vi "Remove Test Property.vi"(6 "timeout (ms)":i32=-1, 8 "error in (no error)":errorcluster, 10 "testPropertyName":string, 11 "FlexLogger_gRPCAPI in":refnum<class "FlexLogger_gRPC.lvclass">) -> (0 "error out":errorcluster, 3 "FlexLogger_gRPCAPI out":refnum<class "FlexLogger_gRPC.lvclass">)   [LabVIEW 2020, in "FlexLogger_gRPC.lvlib" / "FlexLogger_gRPC.lvclass"]
doc: "Removes a specific test property of currently opened project in flexlogger"
uses:
  FlexLogger_gRPC.lvclass
  FlexLogger_client/RPC Messages/flexlogger_RemoveTestPropertyRequest.ctl
  FlexLogger_client/RPC Messages/flexlogger_ElementIdentifier.ctl
  FlexLogger_gRPC.lvclass/FlexLogger_gRPC.ctl
  FlexLogger_client/FlexLogger_client.lvlib
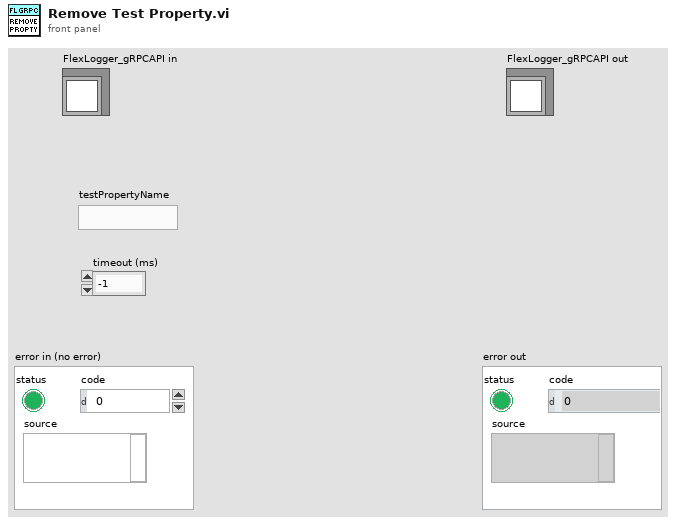
[diagram p1: front panel]
types:
  T1 = typedef "FlexLogger_client.lvlib/flexlogger_RemoveTestPropertyRequest.ctl" = cluster{"document_identifier":T2, "property_name":string}
  T2 = typedef "FlexLogger_client.lvlib/flexlogger_ElementIdentifier.ctl" = cluster{"project_id":string, "file_name":string, "element_id":string, "subpart_id":string}
  T3 = typedef "grpc-lvsupport-release.lvlib/grpcId.ctl" = u64
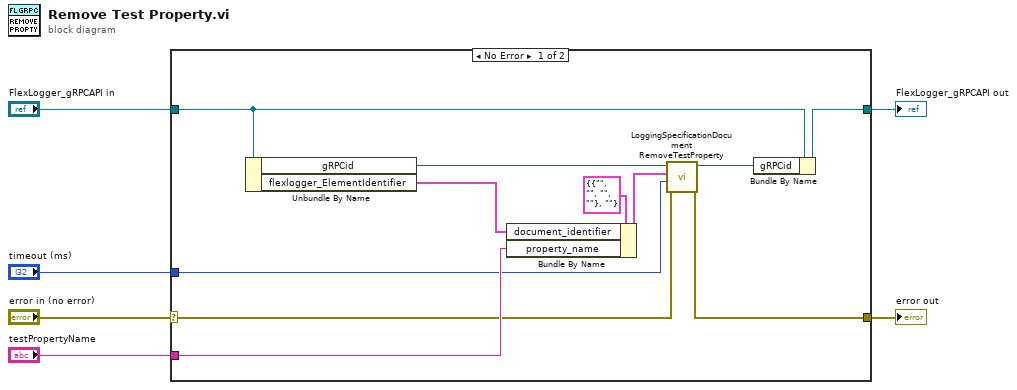
[diagram p0: block diagram]
diagram:
  n1 = case shown="No Error" "error in (no error)" {
    selector: "error in (no error)" -> [w8 w18]
    tunnel: "FlexLogger_gRPCAPI in" -> [w17 w19]
    tunnel: [w16 w19] -> w6
    tunnel: [w13 w18] -> w4
    tunnel: "testPropertyName" -> [w15 _]
    tunnel: "timeout (ms)" -> [w7 _]
    frame No Error {
      n2 = Unbundle By Name(w17) -> ("gRPCid"=w10:T3, "flexlogger_ElementIdentifier"=w9:T2)
      n3 = Bundle By Name(cluster=T1 {"document_identifier"={"project_id"="", "file_name"="", "element_id"="", "subpart_id"=""}, "property_name"=""} ("Request Data"), "document_identifier"=w9, "property_name"=w15) -> (w11:T1)
      n4 = call "LoggingSpecificationDocument RemoveTestProperty.vi"("error in"=w8, "timeout (ms)"=w7, "Request Data"=w11, "gRPC ID"=w10) -> ("error out"=w13:errorcluster, "gRPC ID out"=w14:T3)  [unwired: 5 in, 1 out]
      n5 = Bundle By Name(cluster=w17, "gRPCid"=w14) -> (w16:refnum<class "FlexLogger_gRPC.lvclass">)
    }
    frame Error {
    }
  }
  "error out" <- w4
  "FlexLogger_gRPCAPI out" <- w6
